vi "group_selected_spots.vi"(1 "Selection/Group 2":T1[](array[typedef])) -> (0 "Array":T1[](array[typedef]))   [LabVIEW 2019]
uses:
  selection_element.ctl
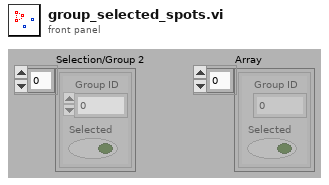
[diagram p1: front panel]
types:
  T1 = typedef "selection_element.ctl" = cluster{"Group ID":i32, "Selected":bool}
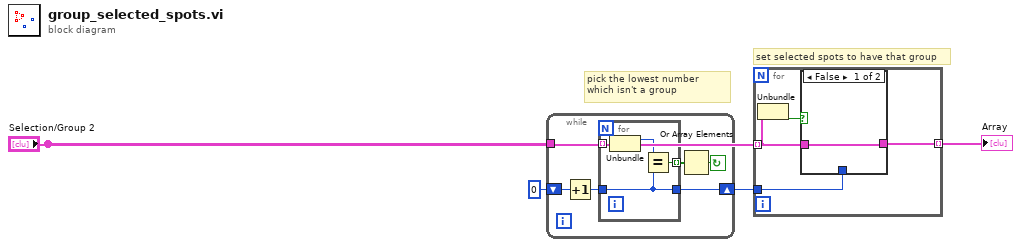
[diagram p0: block diagram]
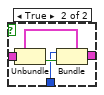
[diagram p2: hidden frame]
diagram:
  # "pick the lowest number which isn't a group"
  # "set selected spots to have that group"
  n1 = while {
    tunnel: "Selection/Group 2" -> [w10]
    shift-right: [w7] -> w1
    shift-left: 0 -> [w6]
    stop <- w9 continue-if-true
    n2 = Increment(x=w6) -> (x+1=w5:i32)
    n3 = for {
      tunnel: w10 -> [w14] mode=indexing
      tunnel: w5 -> [w11]
      tunnel: [w12] -> w8 mode=indexing
      tunnel: [w11] -> w7
      n4 = Unbundle(w14) -> ("Group ID"=w13:i32)  [unwired: 1 out]
      n5 = Equal?(x=w13, y=w11) -> (x = y?=w12:bool)
    }
    n6 = Or Array Elements(Boolean array=w8) -> (logical OR=w9:bool)
  }
  n7 = for {
    tunnel: [w17] -> w3 mode=indexing
    tunnel: "Selection/Group 2" -> [w16] mode=indexing
    tunnel: w1 -> [w15]
    n8 = Unbundle(w16) -> ("Selected"=w18:bool)  [unwired: 1 out]
    n9 = case shown="False" w18 {
      tunnel: [w19 w22] -> w17
      tunnel: w16 -> [w19 w21]
      tunnel: w15 -> [_ w20]
      frame False {
      }
      frame True {
        n10 = Unbundle(w21) -> ("Selected"=w23:bool)  [unwired: 1 out]
        n11 = Bundle(cluster=w21, "Group ID"=w20, "Selected"=w23) -> (w22:T1)
      }
    }
  }
  "Array" <- w3
